vi "SquareInputs.vi"(10 "Square Inputs?":bool, 11 "AxisValueIn":dbl) -> (3 "AxisValueOut":dbl)   [LabVIEW 2013]
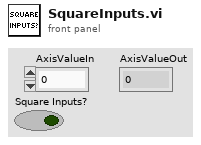
[diagram p1: front panel]
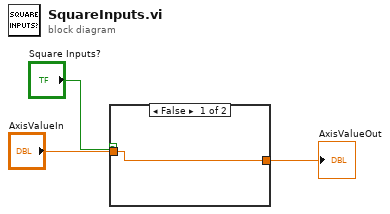
[diagram p0: block diagram]
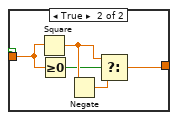
[diagram p2: hidden frame]
diagram:
  n1 = case shown="False" "Square Inputs?" {
    tunnel: [w4 w9] -> w3
    tunnel: "AxisValueIn" -> [w4 w8]
    frame False {
    }
    frame True {
      n2 = Square(x=w8) -> (x^2=w6:dbl)
      n3 = Greater Or Equal To 0?(x=w8) -> (x >= 0?=w5:bool)
      n4 = Negate(x=w6) -> (-x=w7:dbl)
      n5 = Select(t=w6, s=w5, f=w7) -> (s? t:f=w9:dbl)
    }
  }
  "AxisValueOut" <- w3
